vi "File Header Writer.vi"(9 "Data Cluster":T1 {"Amplifier Model" items=["Select a Model", "AM 1700", "BMA 200"]}, 11 "File Path":path) -> (1 "Start Time hr/min":string, 3 "Date mm/dd/yy":string)   [LabVIEW 2014]
uses:
  <vilib>/Utility/file.llb/Write To Spreadsheet File (string).vi
panel:
  # "Inputs"
  # "Outputs"
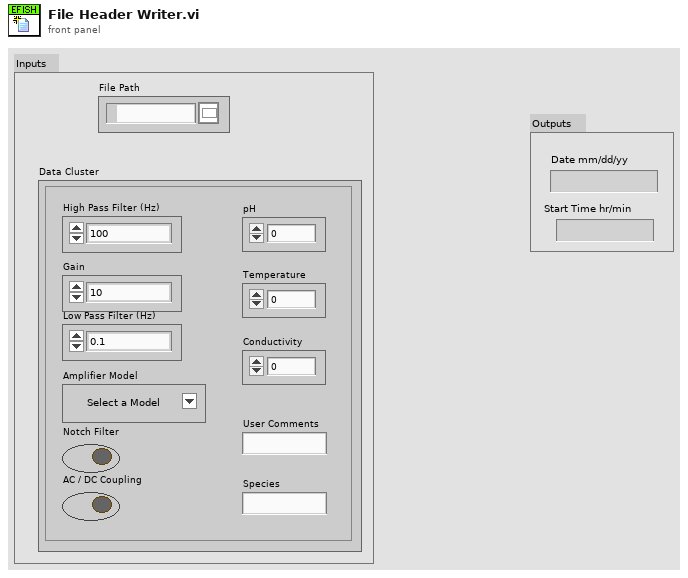
[diagram p1: front panel]
types:
  T1 = cluster{"High Pass Filter (Hz)":enum16{"100", "500", "1000", "3000", "5000", "10,000", "20,000", "30,000", "50,000"}, "Gain":enum16{"10", "20", "50", "100", "200", "500", "1000", "2k", "5k", "10k", "20k", "50k"}, "Low Pass Filter (Hz)":enum16{"0.1", "1", "3", "10", "30", "100", "300"}, "Amplifier Model":u16, "Notch Filter":bool, "AC / DC Coupling":bool, "Temperature":dbl, "Conductivity":dbl, "pH":dbl, "User Comments":string, "Species":string}
  T2 = enum16{"100", "500", "1000", "3000", "5000", "10,000", "20,000", "30,000", "50,000"}
  T3 = enum16{"10", "20", "50", "100", "200", "500", "1000", "2k", "5k", "10k", "20k", "50k"}
  T4 = enum16{"0.1", "1", "3", "10", "30", "100", "300"}
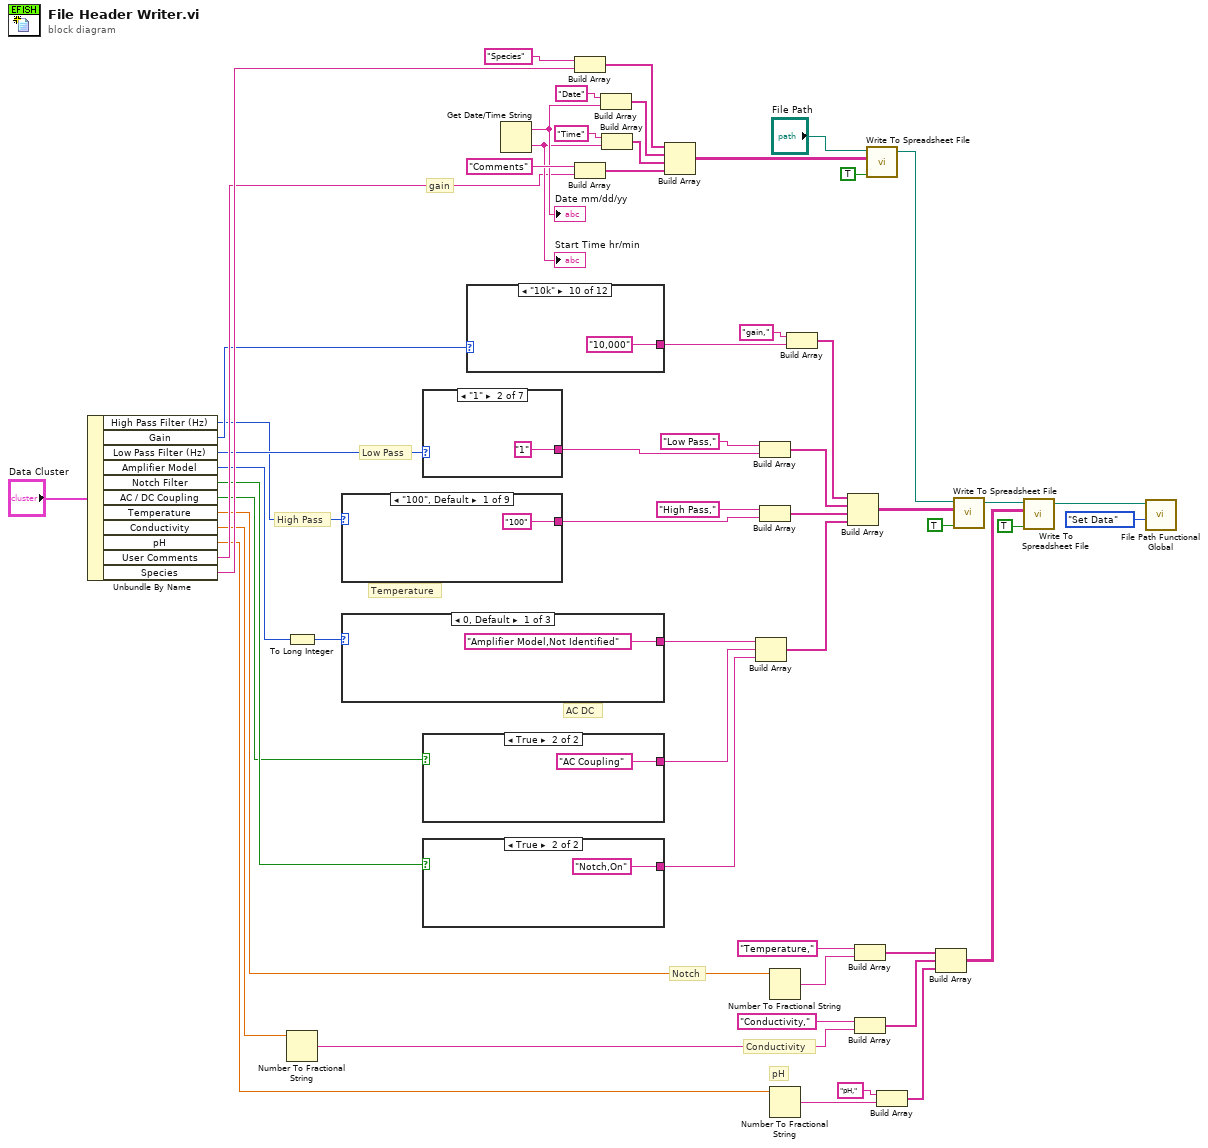
[diagram p0: block diagram]
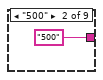
[diagram p2: hidden frame]
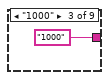
[diagram p3: hidden frame]
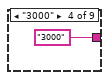
[diagram p4: hidden frame]
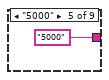
[diagram p5: hidden frame]
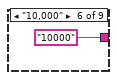
[diagram p6: hidden frame]
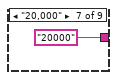
[diagram p7: hidden frame]
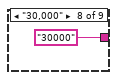
[diagram p8: hidden frame]
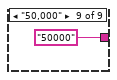
[diagram p9: hidden frame]
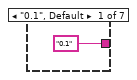
[diagram p10: hidden frame]
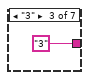
[diagram p11: hidden frame]
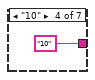
[diagram p12: hidden frame]
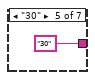
[diagram p13: hidden frame]
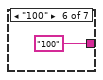
[diagram p14: hidden frame]
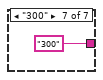
[diagram p15: hidden frame]
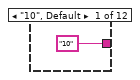
[diagram p16: hidden frame]
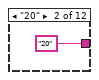
[diagram p17: hidden frame]
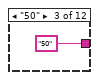
[diagram p18: hidden frame]
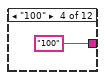
[diagram p19: hidden frame]
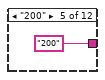
[diagram p20: hidden frame]
diagram:
  # "Low Pass"
  # "pH"
  # "Conductivity"
  # "Temperature"
  # "High Pass"
  # "Notch"
  # "AC DC"
  # "gain"
  n1 = Unbundle By Name("Data Cluster") -> ("High Pass Filter (Hz)"=w9:T2, "Gain"=w12:T3, "Low Pass Filter (Hz)"=w11:T4, "Amplifier Model"=w15:u16, "Notch Filter"=w18:bool, "AC / DC Coupling"=w17:bool, "Temperature"=w19:dbl, "Conductivity"=w20:dbl, "pH"=w21:dbl, "User Comments"=w22:string, "Species"=w23:string)
  n2 = To Long Integer(number=w15) -> (32bit integer=w16:i32)
  n3 = Number To Fractional String(number=w20) -> (F-format string=w33:string)  [unwired: 3 in]
  n4 = case shown="\"100\", Default" w9 {
    tunnel: ["100" "500" "1000" "3000" "5000" "10000" "20000" "30000" "50000"] -> w8
    frame "100", Default {
    }
    frame "500" {
    }
    frame "1000" {
    }
    frame "3000" {
    }
    frame "5000" {
    }
    frame "10,000" {
    }
    frame "20,000" {
    }
    frame "30,000" {
    }
    frame "50,000" {
    }
  }
  n5 = case shown="0, Default" w16 {
    tunnel: ["Amplifier Model,Not Identified" "Model,AM 1700" "Amplify Model,BMA 200"] -> w14
    frame 0, Default {
    }
    frame 1 {
    }
    frame 2 {
    }
  }
  n6 = case shown="\"1\"" w11 {
    tunnel: ["0.1" "1" "3" "10" "30" "100" "300"] -> w10
    frame "0.1", Default {
    }
    frame "1" {
    }
    frame "3" {
    }
    frame "10" {
    }
    frame "30" {
    }
    frame "100" {
    }
    frame "300" {
    }
  }
  n7 = case shown="True" w17 {
    tunnel: ["DC Coupling" "AC Coupling"] -> w38
    frame False {
    }
    frame True {
    }
  }
  n8 = case shown="True" w18 {
    tunnel: ["Notch,Off" "Notch,On"] -> w37
    frame False {
    }
    frame True {
    }
  }
  n9 = case shown="\"10k\"" w12 {
    tunnel: ["10" "20" "50" "100" "200" "500" "1000" "2000" "5000" "10,000" "20,000" "50,000"] -> w13
    frame "10", Default {
    }
    frame "20" {
    }
    frame "50" {
    }
    frame "100" {
    }
    frame "200" {
    }
    frame "500" {
    }
    frame "1000" {
    }
    frame "2k" {
    }
    frame "5k" {
    }
    frame "10k" {
    }
    frame "20k" {
    }
    frame "50k" {
    }
  }
  n10 = Get Date/Time String() -> (date string=w47:string, time string=w46:string)  [unwired: 3 in]
  "Date mm/dd/yy" <- w47
  "Start Time hr/min" <- w46
  n11 = Build Array("Species" ("element"), w23) -> (w51:string[])
  n12 = Build Array("Comments" ("element"), w22) -> (w48:string[])
  n13 = Build Array("Date" ("element"), w47) -> (w50:string[])
  n14 = Build Array("Time" ("element"), w46) -> (w49:string[])
  n15 = Build Array(w51, w50, w49, w48) -> (w6:string[][])
  n16 = Build Array(w14, w38, w37) -> (w36:string[])
  n17 = Build Array("Low Pass," ("string"), w10) -> (w40:string[])
  n18 = Build Array("High Pass," ("string"), w8) -> (w39:string[])
  n19 = Number To Fractional String(number=w19) -> (F-format string=w35:string)  [unwired: 3 in]
  n20 = Number To Fractional String(number=w21) -> (F-format string=w28:string)  [unwired: 3 in]
  n21 = Build Array("gain," ("string"), w13) -> (w41:string[])
  n22 = Build Array(w41, w40, w39, w36) -> (w3:string[][])
  n23 = Build Array("Temperature," ("string"), w35) -> (w32:string[])
  n24 = Build Array("Conductivity," ("string"), w33) -> (w31:string[])
  n25 = call-poly <vilib>:"Write To Spreadsheet File.vi"("append to file? (new file:F)"=TRUE, "2D data"=w6, "file path (dialog if empty)"="File Path") -> ("new file path (Not A Path if cancelled)"=w4:path)  [unwired: 5 in]
  n26 = Build Array("pH," ("element"), w28) -> (w26:string[])
  n27 = Build Array(w32, w31, w26) -> (w29:string[][])
  n28 = call-poly <vilib>:"Write To Spreadsheet File.vi"("append to file? (new file:F)"=TRUE, "2D data"=w3, "file path (dialog if empty)"=w4) -> ("new file path (Not A Path if cancelled)"=w1:path)  [unwired: 5 in]
  n29 = call-poly <vilib>:"Write To Spreadsheet File.vi"("append to file? (new file:F)"=TRUE, "2D data"=w29, "file path (dialog if empty)"=w1) -> ("new file path (Not A Path if cancelled)"=w25:path)  [unwired: 5 in]
  n30 = call "File Path Functional Global.vi"("Enum"=enum16{"Get Data", "Set Data"}."Set Data", "File Path Control"=w25) -> ()  [unwired: 9 in, 1 out]
